vi "cg_Line Minimum Derivative.vi"(6 "tol":dbl=1e-06 format="%.2e", 7 "function and data":T1, 8 "error in (no error)":errorcluster, 9 "p":dbl[](array[numeric]) format="%.2f", 11 "xit":dbl[](array[numeric]) format="%.2f") -> (0 "error out":errorcluster, 1 "f(p)":dbl format="%.2f", 2 "pnew":dbl[](array[numeric]) format="%.2f", 3 "xitnew":dbl[](array[numeric]) format="%.2f", 5 "number of function evaluations":i32)   [LabVIEW 2018, in "NI_Gmath.lvlib"]
uses:
  NI_Gmath.lvlib
  ucno_user function ref and data.ctl
  ucno_user objective function ref.ctl
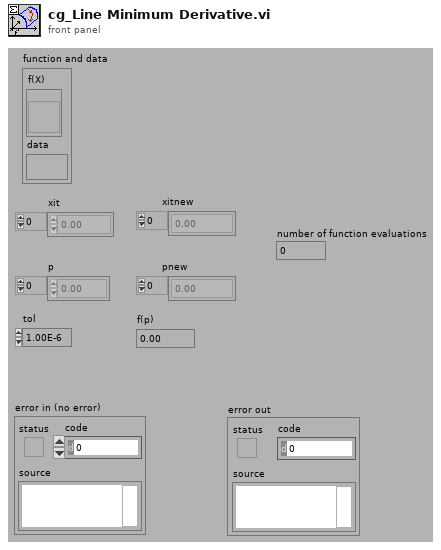
[diagram p1: front panel]
types:
  T1 = typedef "NI_Gmath.lvlib/ucno_user function ref and data.ctl" = cluster{"f(X)":T2, "data":variant}
  T2 = typedef "NI_Gmath.lvlib/ucno_user objective function ref.ctl" = refnum<vi>
  T3 = cluster{"objective function":bool, "gradient":bool}
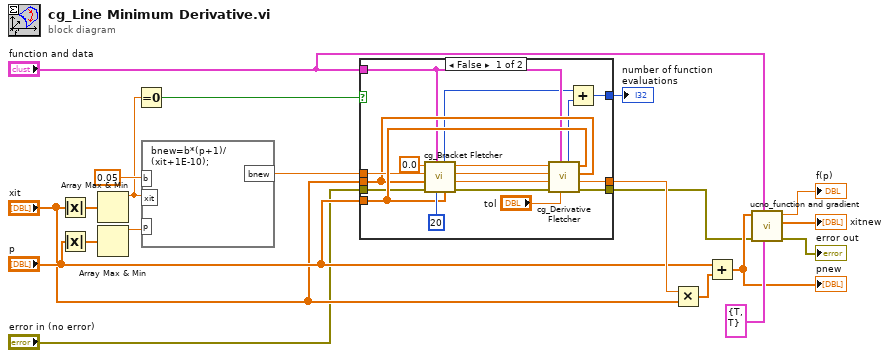
[diagram p0: block diagram]
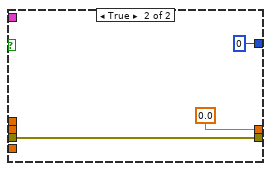
[diagram p2: hidden frame]
diagram:
  n1 = Absolute Value(x="xit") -> (abs(x)=w12:dbl[])
  n2 = Absolute Value(x="p") -> (abs(x)=w11:dbl[])
  n3 = Array Max & Min(array=w12) -> (max value=w8:dbl)  [unwired: 3 out]
  n4 = Array Max & Min(array=w11) -> (max value=w9:dbl)  [unwired: 3 out]
  n5 = Equal To 0?(x=w8) -> (x = 0?=w7:bool)
  n6 = formula code="bnew=b*(p+1)/(xit+1E-10);"("b"=0.05, "xit"=w8, "p"=w9) -> ("bnew"=w14:dbl)
  n7 = case shown="False" w7 {
    tunnel: "p" -> [w35 _]
    tunnel: w14 -> [w34 _]
    tunnel: [w33 0.0] -> w15
    tunnel: "xit" -> [w28 _]
    tunnel: [w26 w39] -> w5
    tunnel: "error in (no error)" -> [w25 w39]
    tunnel: "function and data" -> [w24 _]
    tunnel: [w21 0] -> w1
    frame False {
      n8 = call "cg_Bracket Fletcher.vi"("p"=w35, "loops"=u32 20, "function and data"=w24, "error in (no error)"=w25, "xit"=w28, "b (start)"=w34, "a (start)"=0.0) -> ("error out"=w27:errorcluster, "c (bracket)"=w32:dbl, "b (bracket)"=w31:dbl, "a (bracket)"=w30:dbl, "number of function calls"=w22:i32)
      n9 = call "cg_Derivative Fletcher.vi"("xi"=w28, "p"=w35, "ftol"="tol", "function and data"=w24, "error in (no error)"=w27, "c (start)"=w32, "b (start)"=w31, "a (start)"=w30) -> ("error out"=w26:errorcluster, "x"=w33:dbl, "number of function calls"=w23:i32)  [unwired: 1 out]
      n10 = Add(x=w22, y=w23) -> (x+y=w21:i32)
    }
    frame True {
    }
  }
  "number of function evaluations" <- w1
  n11 = Multiply(x=w15, y="xit") -> (x*y=w17:dbl[])
  n12 = Add(x="p", y=w17) -> (x+y=w19:dbl[])
  "pnew" <- w19
  n13 = call "ucno_function and gradient.vi"("output control"=T3 {"objective function"=TRUE, "gradient"=TRUE}, "function and data"="function and data", "error in (no error)"=w5, "X"=w19) -> ("error out"=→"error out":errorcluster, "gradient"=→"xitnew":dbl[], "f(X)"=→"f(p)":dbl)  [unwired: 4 in, 1 out]
